vi "closeThreads.vi"() -> ()   [LabVIEW 2020]
panel:
  out "Stop thread temp":bool
  out "Stop acquisition":bool
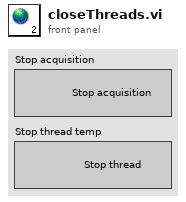
[diagram p1: front panel]
diagram:
